vi "Panel RMC Calculator.vi"(0 "Scale Com Port":refnum<visa-resource-name>="COM1", 5 "Bone Dry Wt(lbs)":dbl=7.0 format="%03_6g") -> (6 "Weights Out":T1={"Measured IMC"=7.0, "Actual RMC"=7.0, "RMC (Desired)"=100.0, "Bone Dry Wt(lbs)"=7.0, "Tolerance(%)"=5.0} {"Tolerance(%)" format="%0#_6g"; "Bone Dry Wt(lbs)" format="%03_6g"; "RMC (Desired)" format="%0#_6g"; "Actual RMC" format="%03_6g"; "Measured IMC" format="%0#_6g"})   [LabVIEW 2012]
panel:
  in  "Read Scale for IMC":bool
  out "Actual RMC":dbl=7.0 format="%03_6g"
  in  "Measured IMC (lbs)":dbl=7.0 format="%0#_6g"
  in  "Tolerance(%)":dbl=5.0 format="%0#_6g"
  in  "RMC (Desired)":dbl format="%0#_6g"
  out "Nominal":dbl=7.0 format="%03_6g"
  out "Min":dbl=7.0 format="%03_6g"
  out "Max":dbl=7.0 format="%03_6g"
  in  "stop":bool
  # "RMC Calculator"
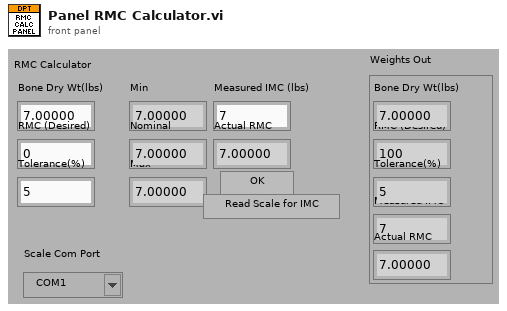
[diagram p1: front panel]
types:
  T1 = cluster{"Measured IMC":dbl, "Actual RMC":dbl, "RMC (Desired)":dbl, "Bone Dry Wt(lbs)":dbl, "Tolerance(%)":dbl}
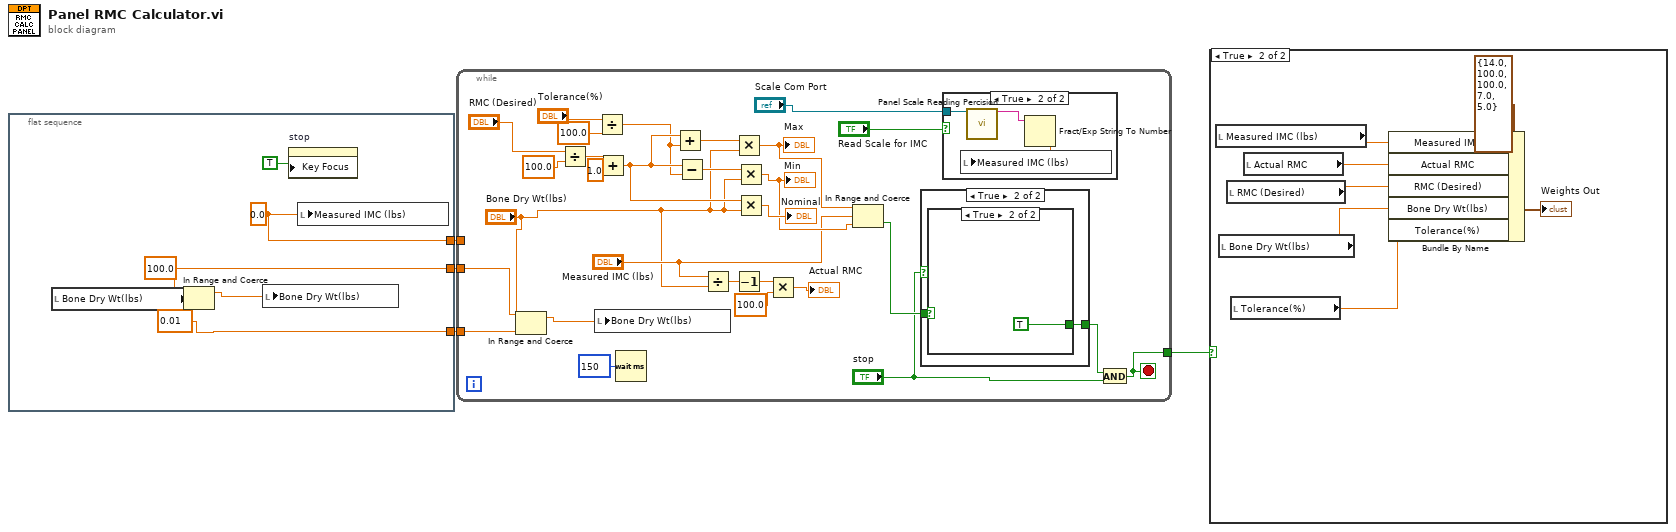
[diagram p0: block diagram]
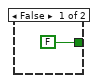
[diagram p4: hidden frame]
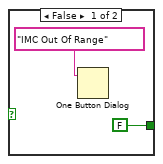
[diagram p5: hidden frame]
diagram:
  n1 = flat-sequence {
    tunnel: [w10] -> w4
    tunnel: [w7] -> w2
    tunnel: [w6] -> w1
    frame #0 {
      w7 = 100.0 ("upper limit")
      w6 = 0.01 ("lower limit")
      w10 = 0.0 ("Measured IMC(Initial Moisture Content)")
      n2 = local read "Bone Dry Wt(lbs)"() -> (w9:dbl)
      n3 = In Range and Coerce(upper limit=w7, x=w9, lower limit=w6) -> (coerced(x)=w8:dbl)  [unwired: 1 out]
      n4 = local write "Bone Dry Wt(lbs)"(w8) -> ()
      n5 = property on="stop" class="Bool"("Key Focus"=TRUE) -> ()  [unwired: 2 in, 2 out]
      n6 = local write "Measured IMC (lbs)"(w10) -> ()
    }
  }
  n7 = while {
    tunnel: w4 -> [_]
    tunnel: [w17] -> w3
    tunnel: w2 -> [w14]
    tunnel: w1 -> [w13]
    stop <- w17 stop-if-true
    n8 = In Range and Coerce(upper limit=w14, x="Bone Dry Wt(lbs)", lower limit=w13) -> (coerced(x)=w16:dbl)  [unwired: 1 out]
    n9 = Divide(x="RMC (Desired)", y=100.0) -> (x/y=w34:dbl)
    n10 = local write "Bone Dry Wt(lbs)"(w16) -> ()
    n11 = Divide(x="Tolerance(%)", y=100.0) -> (x/y=w29:dbl)
    n12 = Add(x=w34, y=1.0) -> (x+y=w31:dbl)
    n13 = Wait (ms)(milliseconds to wait=u32 150) -> ()  [unwired: 1 out]
    n14 = Add(x=w31, y=w29) -> (x+y=w36:dbl)
    n15 = Subtract(x=w31, y=w29) -> (x-y=w37:dbl)
    n16 = Divide(x="Measured IMC (lbs)", y="Bone Dry Wt(lbs)") -> (x/y=w21:dbl)
    n17 = Multiply(x=w36, y="Bone Dry Wt(lbs)") -> (x*y=w26:dbl)
    "Max" <- w26
    n18 = Decrement(x=w21) -> (x-1=w19:dbl)
    n19 = Multiply(x=w37, y="Bone Dry Wt(lbs)") -> (x*y=w25:dbl)
    "Min" <- w25
    n20 = Multiply(x=w31, y="Bone Dry Wt(lbs)") -> (x*y=→"Nominal":dbl)
    n21 = Multiply(x=w19, y=100.0 ("x-1")) -> (x*y=→"Actual RMC":dbl)
    n22 = In Range and Coerce(upper limit=w26, x="Measured IMC (lbs)", lower limit=w25) -> (In Range?=w27:bool)  [unwired: 1 out]
    n23 = case shown="True" "stop" {
      tunnel: w27 -> [_ w45]
      tunnel: [FALSE w44] -> w24
      frame False {
      }
      frame True {
        n24 = case shown="True" w45 {
          tunnel: [FALSE TRUE] -> w44
          frame False {
            n25 = One Button Dialog(message="IMC Out Of Range") -> ()  [unwired: 1 in, 1 out]
          }
          frame True {
          }
        }
      }
    }
    n26 = case shown="True" "Read Scale for IMC" {
      tunnel: "Scale Com Port" -> [_ w40]
      frame False {
      }
      frame True {
        n27 = call "Panel Scale Reading Percision.vi"("VISA resource name"=w40) -> ("read buffer"=w42:string)  [unwired: 14 in]
        n28 = Fract/Exp String To Number(string=w42) -> (number=w41:dbl)  [unwired: 3 in, 1 out]
        n29 = local write "Measured IMC (lbs)"(w41) -> ()
      }
    }
    n30 = And(x=w24, y="stop") -> (x .and. y?=w17:bool)
  }
  n31 = case shown="True" w3 {
    frame False {
    }
    frame True {
      n32 = local read "Measured IMC (lbs)"() -> (w55:dbl)
      n33 = local read "Bone Dry Wt(lbs)"() -> (w52:dbl)
      n34 = local read "RMC (Desired)"() -> (w53:dbl)
      n35 = local read "Tolerance(%)"() -> (w51:dbl)
      n36 = local read "Actual RMC"() -> (w54:dbl)
      n37 = Bundle By Name(cluster=T1 {"Measured IMC"=14.0, "Actual RMC"=100.0, "RMC (Desired)"=100.0, "Bone Dry Wt(lbs)"=7.0, "Tolerance(%)"=5.0} ("Weights Out"), "Measured IMC"=w55, "Actual RMC"=w54, "RMC (Desired)"=w53, "Bone Dry Wt(lbs)"=w52, "Tolerance(%)"=w51) -> (→"Weights Out":T1)
    }
  }
